vi "Voice.vi"(4 "Run / Stop":refnum<vi>, 5 "Event Data":cluster{"sender":refnum<k24>, "e":refnum<k24>}, 6 "Control Ref":refnum<k24>, 7 "Event Common Data":T1) -> ()   [LabVIEW 2014]
uses:
  System.Speech
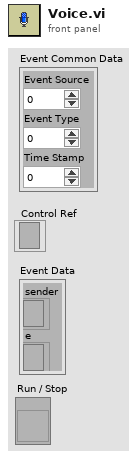
[diagram p1: front panel]
types:
  T1 = cluster{"Event Source":i32, "Event Type":u32, "Time Stamp":u32}
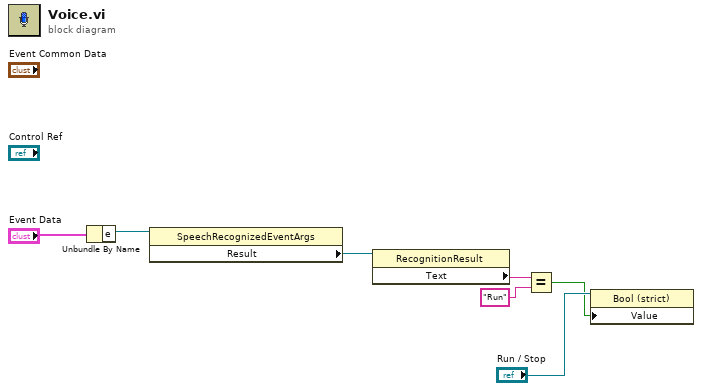
[diagram p0: block diagram]
diagram:
  n1 = Unbundle By Name("Event Data") -> ("e"=w6:refnum<k24>)
  n2 = property class="SpeechRecognizedEventArgs"(reference=w6) -> ("Result"=w5:refnum<k24>)  [unwired: 1 in, 2 out]
  n3 = property class="RecognitionResult"(reference=w5) -> ("Text"=w3:string)  [unwired: 1 in, 2 out]
  n4 = Equal?(x=w3, y="Run") -> (x = y?=w1:bool)
  n5 = property class="Bool (strict)"(reference="Run / Stop", "Value"=w1) -> ()  [unwired: 1 in, 2 out]
